vi "MUX RT Driver VI.vi"(6 "Device Clock":string, 9 "Device Inputs FIFO":refnum<k33>, 10 "Device Outputs FIFO":refnum<k33>, 11 "Device Reference":T1 format="%.0x") -> ()   [LabVIEW 2013, in "MUX Custom Device.lvlib"]
uses:
  MUX Custom Device.lvlib
  <vilib>/NI Veristand/Custom Device API/Custom Device Item Ref.ctl
  <vilib>/NI Veristand/Custom Device API/Custom Device Channel Type.ctl
  <vilib>/Platform/TimedLoop/XDataNode/timing_clust.ctl
  <vilib>/Platform/TimedLoop/XDataNode/nitl_modes.ctl
  <vilib>/Platform/TimedLoop/XDataNode/wakeup.ctl
  <instrlib>/niSwitch/niSwitch.LLB/niSwitch Relay Action.ctl
  MUX Global.vi
  <vilib>/NI Veristand/Custom Device API/Get Item Property (String).vi
  <vilib>/Platform/TimedLoop/XDataNode/XDataNode.xnode
  <vilib>/Platform/TimedLoop/XDataNode/XDNodeRunTimeDep.lvlib
  <vilib>/NI Veristand/Custom Device API/Custom Device API.lvlib
  <vilib>/NI Veristand/Custom Device Tools/Custom Device Utility Library/Custom Device Utility Library.lvlib
panel:
  in  "Status Notifier":refnum<notifier>
  # "Custom Device Template\nv1.0"
  # "Use this template as a starting point for creating a custom device code module. The input controls shown here are specially named controls that the system will use to provide the device loop with data. The controls are not required for the device loop to run. For instance, if the device doesn't produce any output data, then you don't need the Device Outputs FIFO control. If you do use these controls, however, they need to have these exact names to be functional."
  # "The optional status notifier element is used to notify the RT engine of the last state of the custom device, and to indicate the device has completed execution. If this control is not used, a default No Error value is returned to the system when the device finishes execution.\n\nNote: This error state is not checked until the system shuts down. Use an output status channel to send more immediate status values to the system."
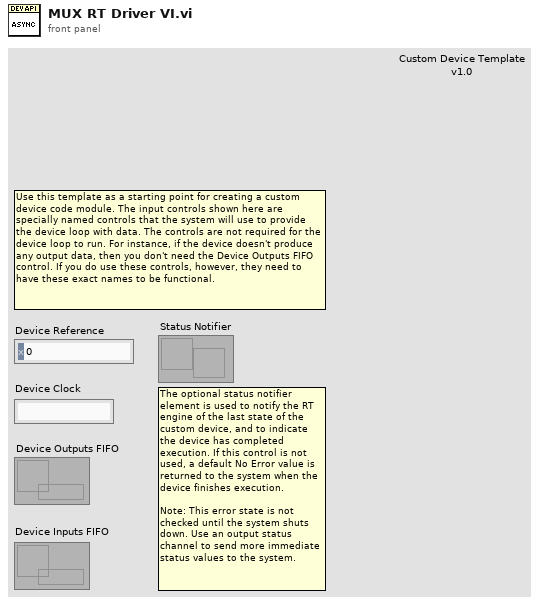
[diagram p1: front panel]
types:
  T1 = typedef "Custom Device API.lvlib/Custom Device Item Ref.ctl" = u64
  T2 = typedef "Custom Device API.lvlib/Custom Device Channel Type.ctl" = enum16{"Input", "Output"}
  T3 = typedef "Custom Device API.lvlib/Custom Device Timed Loop Priority.ctl" = enum32{"Low", "Medium", "High"}
  T4 = typedef "XDNodeRunTimeDep.lvlib/timing_clust.ctl" = cluster{"Expected End [f-1]":u64, "Actual End [f-1]":u64, "Finished Late? [f-1]":bool, "Expected End [i-1]":u64, "Actual End [i-1]":u64, "Finished Late? [i-1]":bool, "Expected Start [i]":u64, "Actual Start [i]":u64, "Expected Start [f]":u64, "Actual Start [f]":u64, "Source Name":string, "Structure Name":string, "Period":i64, "Deadline":i64, "Offset":i64, "Start":i64, "Priority":i32, "Timeout":i32, "Mode":T5, "Wakeup Reason":T6, "Error":errorcluster, "Source Type":string, "Secondary Source Type":string, "Global End Time":u64, "Global Start Time":u64, "Frame Duration":u64, "Iteration Duration":u64, "Assigned CPU":i32, "I/O Scan Engine Mode":u32}
  T5 = typedef "XDNodeRunTimeDep.lvlib/nitl_modes.ctl" = enum32{"No Change", "Process missed periods, maintain original phase", "Discard missed periods, maintain original phase", "Process missed periods, ignore original phase", "Discard missed periods, ignore original phase"}
  T6 = typedef "XDNodeRunTimeDep.lvlib/wakeup.ctl" = enum32{"Normal", "Aborted", "Asynchronous wakeup", "Timing source error", "Timed loop error", "Timeout"}
  T7 = typedef "niSwitch Relay Action.ctl" = i32
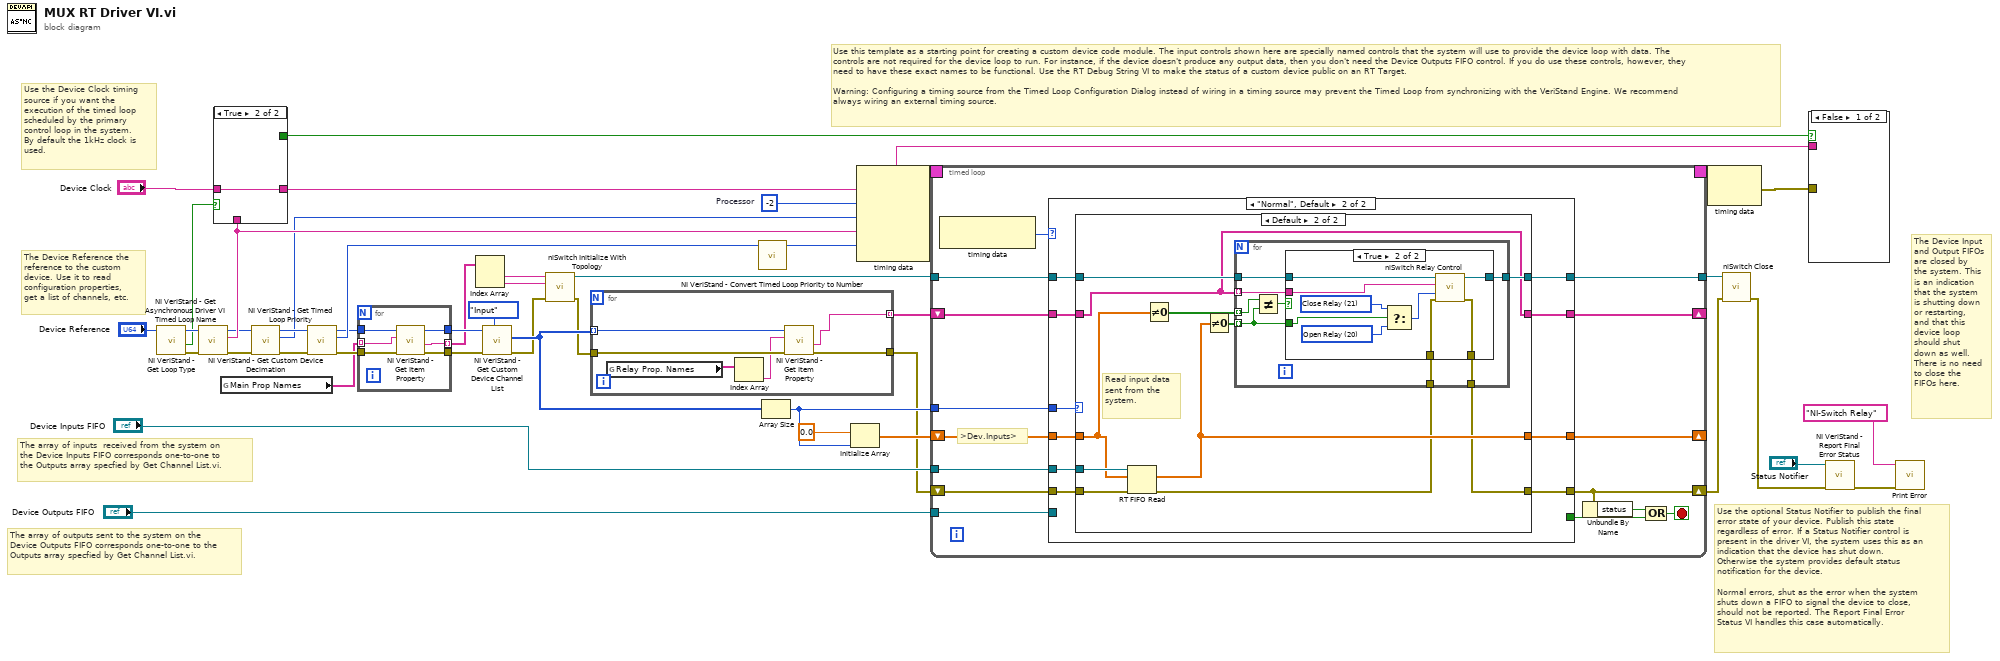
[diagram p0: block diagram]
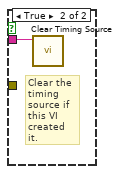
[diagram p2: hidden frame]
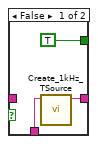
[diagram p3: hidden frame]
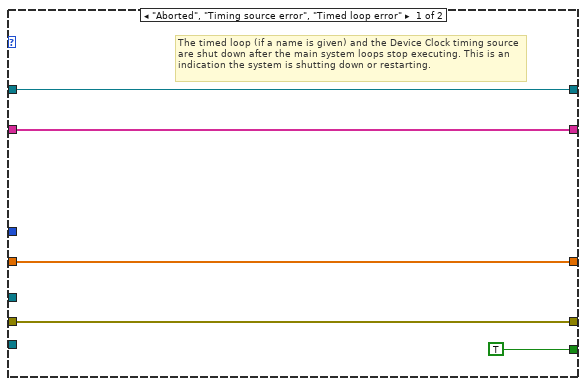
[diagram p4: hidden frame]
diagram:
  w36 = -2  # Processor
  # "The array of inputs  received from the system on the Device Inputs FIFO corresponds one-to-one to the Outputs array specfied by Get Channel List.vi."
  # "Use the optional Status Notifier to publish the final error state of your device. Publish this state regardless of error. If a Status Notifier control is present in the driver VI, the system uses this as an indication that the device has shut down. Otherwise the system provides default status notification for the device.\n\nNormal errors, shut as the error when the system shuts down a FIFO to signal the device to close, should not be reported. The Report Final Error Status VI handles this case automatically."
  # "The Device Input and Output FIFOs are closed by the system. This is an indication that the system is shutting down or restarting, and that this device loop should shut down as well. There is no need to close the FIFOs here."
  # "The array of outputs sent to the system on the Device Outputs FIFO corresponds one-to-one to the Outputs array specfied by Get Channel List.vi."
  # "The Device Reference the reference to the custom device. Use it to read configuration properties, get a list of channels, etc."
  # "Use the Device Clock timing source if you want the execution of the timed loop scheduled by the primary control loop in the system. \nBy default the 1kHz clock is used."
  # "Use this template as a starting point for creating a custom device code module. The input controls shown here are specially named controls that the system will use to provide the device loop with data. The controls are not required for the device loop to run. For instance, if the device doesn't produce any output data, then you don't need the Device Outputs FIFO control. If you do use these controls, however, they need to have these exact names to be functional. Use the RT Debug String VI to make the status of a custom device public on an RT Target.\n\nWarning: Configuring a timing source from the Timed Loop Configuration Dialog instead of wiring in a timing source may prevent the Timed Loop from synchronizing with the VeriStand Engine. We recommend always wiring an external timing source."
  n1 = call <vilib>:"NI VeriStand - Get Loop Type.vi"("Device Ref in"="Device Reference") -> ("error out"=w34:errorcluster, "Use Device Clock"=w31:bool, "Device Ref out"=w33:T1)  [unwired: 1 in, 7 out]
  n2 = call <vilib>:"NI VeriStand - Get Asynchronous Driver VI Timed Loop Name.vi"("error in (no error)"=w34, "Device Ref in"=w33) -> ("error out"=w22:errorcluster, "Device Timed Loop Name"=w25:string, "Device Ref out"=w24:T1)  [unwired: 7 out]
  n3 = case shown="True" w31 {
    tunnel: "Device Clock" -> [_ w49]
    tunnel: [w48 w49] -> w26
    tunnel: [TRUE _] -> w27
    tunnel: w25 -> [w46 _]
    frame False {
      n4 = call <vilib>:"Create_1kHz_TSource.vi"("name (in)"=w46) -> ("name (out)"=w48:string)  [unwired: 1 in, 9 out]
    }
    frame True {
    }
  }
  n5 = global read "MUX Global.vi" "Main Prop Names"() -> (w12:string[])
  n6 = call <vilib>:"NI VeriStand - Get Custom Device Decimation.vi"("error in (no error)"=w22, "Device Ref in"=w24) -> ("error out"=w21:errorcluster, "Decimation"=w20:i32, "Device Ref out"=w23:T1)  [unwired: 7 in]
  n7 = call <vilib>:"NI VeriStand - Get Timed Loop Priority.vi"("error in (no error)"=w21, "Device Ref in"=w23) -> ("error out"=w16:errorcluster, "Priority"=w38:T3, "Device Ref out"=w15:T1)  [unwired: 7 out]
  n8 = for {
    tunnel: w16 -> [w55]
    tunnel: w15 -> [w54]
    tunnel: [w53] -> w14
    tunnel: [w52] -> w13
    tunnel: w12 -> [w51] mode=indexing
    tunnel: [w50] -> w11 mode=indexing
    n9 = call-poly <vilib>:"NI VeriStand - Get Item Property.vi"("error in (no error)"=w55, "Property Name"=w51, "Item Ref in"=w54) -> ("error out"=w52:errorcluster, "Value"=w50:string, "Item Ref out"=w53:T1)  [unwired: 5 in, 1 out]
  }
  n10 = Index Array(array=w11) -> (element #1=w10:string, element #2=w9:string)  [unwired: 2 in]
  n11 = call <vilib>:"NI VeriStand - Get Custom Device Channel List.vi"("Channel Type"=Custom_Device_Channel_Type."Input", "error in (no error)"=w13, "Device Ref in"=w14) -> ("error out"=w5:errorcluster, "Specified Channel Ref List"=w19:T1[])  [unwired: 7 out]
  n12 = call <instrlib>:"niSwitch Initialize With Topology.vi"("error in (no error)"=w5, "topology name"=w9, "resource name"=w10) -> ("error out"=w4:errorcluster, "instrument handle out"=w6:refnum<k15>)  [unwired: 7 in]
  n13 = for {
    tunnel: w19 -> [w61] mode=indexing
    tunnel: w4 -> [w60]
    tunnel: [w56] -> w18
    tunnel: [w57] -> w17 mode=indexing
    n14 = global read "MUX Global.vi" "Relay Prop. Names"() -> (w59:string[])
    n15 = Index Array(array=w59) -> (element=w58:string)  [unwired: 1 in]
    n16 = call-poly <vilib>:"NI VeriStand - Get Item Property.vi"("error in (no error)"=w60, "Property Name"=w58, "Item Ref in"=w61) -> ("error out"=w56:errorcluster, "Value"=w57:string)  [unwired: 5 in, 2 out]
  }
  n17 = call <vilib>:"NI VeriStand - Convert Timed Loop Priority to Number.vi"("Priority"=w38) -> ("Numeric Priority"=w37:i32)  [unwired: 10 out]
  n18 = Array Size(array=w19) -> (size(s)=w35:i32)
  n19 = Initialize Array(0.0 ("element"), w35) -> (w40:dbl[])
  n20 = node-c288(w26, w36, w20, w25, w37) -> (w43:T4)
  n21 = timed-loop {
    timing: w43 -> [_]
    timing-out: [_] -> w42
    shift-right: [w74] -> _
    shift-left: w40 -> [w75]
    shift-right: [w70] -> w8
    shift-left: w18 -> [w76]
    tunnel: "Device Outputs FIFO" -> [w72]
    tunnel: "Device Inputs FIFO" -> [w71]
    tunnel: w35 -> [w66]
    shift-right: [w64] -> _
    shift-left: w17 -> [w65]
    tunnel: [w63] -> w7
    tunnel: w6 -> [w62]
    stop <- w67 stop-if-true
    # ">Dev.Inputs>"
    n22 = node-c288() -> (w73:T6)  [unwired: 1 out]
    n23 = case shown="\"Normal\", Default" w73 {
      tunnel: w76 -> [w80 w89]
      tunnel: w75 -> [w81 w90]
      tunnel: [w80 w85] -> w70
      tunnel: [w81 w86] -> w74
      tunnel: w72 -> [_ _]
      tunnel: w71 -> [_ w91]
      tunnel: [TRUE _] -> w68
      tunnel: w66 -> [_ w88]
      tunnel: w65 -> [w78 w87]
      tunnel: [w78 w84] -> w64
      tunnel: [w77 w83] -> w63
      tunnel: w62 -> [w77 w82]
      frame "Aborted", "Timing source error", "Timed loop error" {
        # "The timed loop (if a name is given) and the Device Clock timing source are shut down after the main system loops stop executing. This is an indication the system is shutting down or restarting."
      }
      frame "Normal", Default {
        n24 = case shown="Default" w88 {
          tunnel: w91 -> [_ w106]
          tunnel: w90 -> [w95 w97]
          tunnel: [w95 w104] -> w86
          tunnel: [w94 w100] -> w85
          tunnel: w89 -> [w94 w105]
          tunnel: w87 -> [w93 w98]
          tunnel: [w93 w98] -> w84
          tunnel: [w92 w103] -> w83
          tunnel: w82 -> [w92 w102]
          frame 0 {
            # "No inputs to read\nfrom system. Inputs FIFO not created in this case, so don't write to it."
          }
          frame Default {
            # "Read input data sent from the system."
            n25 = RT FIFO Read(0:w106, 1:w97, 3:w105) -> (9:w104:dbl[], 11:w101:errorcluster)  [unwired: 4 out]
            n26 = Not Equal To 0?(x=w97) -> (x != 0?=w96:bool[])
            n27 = Not Equal To 0?(x=w104) -> (x != 0?=w99:bool[])
            n28 = for {
              tunnel: [w114] -> w103
              tunnel: w102 -> [w113]
              tunnel: w101 -> [w112]
              tunnel: [w111] -> w100
              tunnel: w99 -> [w108] mode=indexing
              tunnel: w98 -> [w110] mode=indexing
              tunnel: w96 -> [w109] mode=indexing
              n29 = Not Equal?(x=w109, y=w108) -> (x != y?=w107:bool)
              n30 = case shown="True" w107 {
                tunnel: [w116 w125] -> w114
                tunnel: w113 -> [w116 w124]
                tunnel: w112 -> [w115 w123]
                tunnel: [w115 w122] -> w111
                tunnel: w108 -> [_ w119]
                tunnel: w110 -> [_ w117]
                frame False {
                }
                frame True {
                  w121 = T7 20 items=["Open Relay"=20, "Close Relay"=21] ("relay action (Close Relay)")
                  w120 = T7 21 items=["Open Relay"=20, "Close Relay"=21] ("relay action (Close Relay)")
                  n31 = Select(t=w120, s=w119, f=w121) -> (s? t:f=w118:T7)
                  n32 = call <instrlib>:"niSwitch Relay Control.vi"("error in (no error)"=w123, "relay action (Close Relay)"=w118, "relay name"=w117, "instrument handle"=w124) -> ("error out"=w122:errorcluster, "instrument handle out"=w125:refnum<k15>)  [unwired: 6 in]
                }
              }
            }
          }
        }
      }
    }
    n33 = Unbundle By Name(w70) -> ("status"=w69:bool)
    n34 = Compound Arithmetic op=OR(w69, w68) -> (w67:bool)
  }
  n35 = node-c288(w42) -> (w28:errorcluster)
  n36 = call <instrlib>:"niSwitch Close.vi"("error in (no error)"=w8, "instrument handle"=w7) -> ("error out"=w3:errorcluster)  [unwired: 9 in]
  n37 = case shown="False" w27 {
    tunnel: w28 -> [_ _]
    tunnel: w26 -> [_ w129]
    frame False {
    }
    frame True {
      # "Clear the timing source if this VI created it."
      n38 = call <vilib>:"Clear Timing Source.vi"("name"=w129) -> ()  [unwired: 1 in, 10 out]
    }
  }
  n39 = call <vilib>:"NI VeriStand - Report Final Error Status.vi"("error in (no error)"=w3, "Status Notifier"="Status Notifier") -> ("error out"=w2:errorcluster)  [unwired: 1 in, 8 out]
  n40 = call "Print Error.vi"("error out"=w2, "Your code's public name"="NI-Switch Relay") -> ()  [unwired: 9 in]
